vi "eserc_4_lettura.vi"() -> ()   [LabVIEW 2021]
uses:
  DMM4.lvlib
panel:
  out "CORRENTE":dbl[](array[numeric])=[2.0202, 2.0202, 2.0202, 2.0202, 2.0203, 2.0203, 2.0203, 2.0203, 2.0203, 2.0203, 2.0203, 2.0203, 2.0203, 2.0203, 2.0203, 2.0203, 2.0203, 2.0203, 2.0203, 2.0203, 2.0203, 2.0203, 2.0203, 2.0203, 2.0203, 2.0203, 2.0203, 2.0203, 2.0203, 2.0203, 2.0203, 2.0203, 2.0203, 2.0203, 2.0203, 2.0203, 2.0203, 2.0203, 2.0203, 2.0203, 2.0203, 2.0203, 2.0203, 2.0203, 2.0203, 2.0203, 2.0203, 2.0203, 2.0203, 2.0203, 2.0203, 2.0203, 2.0203, 2.0203, 2.0203, 2.0203, 2.0203, 2.0203, 2.0203, 2.0203, 2.0203, 2.0203, 2.0203, 2.0203, 2.0203, 2.0203, 2.0203, 2.0203, 2.0203, 2.0203, 2.0203, 2.0203, 2.0203, 2.0203, 2.0203, 2.0203, 2.0203, 2.0203, 2.0203, 2.0203, 2.0203, 2.0203, 2.0203, 2.0203, 2.0203, 2.0203, 2.0203, 2.0203, 2.0203, 2.0203, 2.0203, 2.0203, 2.0203, 2.0203, 2.0203, 2.0203, 2.0203, 2.0203, 2.0203, 2.0203]
  out "TENSIONE":dbl[](array[numeric])=[0.00906, 0.00906, 0.00906, 0.00906, 0.00906, 0.00906, 0.00906, 0.00906, 0.00906, 0.00906, 0.00906, 0.00906, 0.00906, 0.00906, 0.00906, 0.00906, 0.00906, 0.00906, 0.00906, 0.00906, 0.00906, 0.00906, 0.00906, 0.00906, 0.00906, 0.00906, 0.00906, 0.00906, 0.00906, 0.00906, 0.00906, 0.00906, 0.00906, 0.00905, 0.00905, 0.00905, 0.00906, 0.00906, 0.00906, 0.00906, 0.00905, 0.00905, 0.00905, 0.00906, 0.00906, 0.00906, 0.00906, 0.00906, 0.00906, 0.00906, 0.00905, 0.00905, 0.00905, 0.00905, 0.00906, 0.00905, 0.00906, 0.00906, 0.00906, 0.00906, 0.00905, 0.00906, 0.00906, 0.00906, 0.00906, 0.00906, 0.00905, 0.00905, 0.00905, 0.00905, 0.00906, 0.00906, 0.00906, 0.00906, 0.00906, 0.00905, 0.00905, 0.00906, 0.00905, 0.00905, 0.00905, 0.00905, 0.00905, 0.00905, 0.00905, 0.00905, 0.00905, 0.00905, 0.00905, 0.00906, 0.00905, 0.00905, 0.00905, 0.00905, 0.00905, 0.00906, 0.00905, 0.00905, 0.00905, 0.00906]
  in  "BOTTONE A":bool
  in  "BOTTONE V":bool
  out "error out 2":errorcluster
  out "Measure Value 2":string="+2.0203E+0\r\n"
  in  "Stop 2":bool
  out "Boolean 2":bool=TRUE
  in  "Detector Rate 2":u16(ring) items=["SLOW", "MID", "FAST"]
  in  "Manual Range 2":dbl=5.0 format="%#.9e"
  in  "Enable Auto Range 2":bool
  out "ID Return String 2":string="GWInstek,GDM8341,GEP843370,1.03\r\n"
  in  "Configure RS232 Baud Rate 2":u32(ring)=115200 items=["9600"=9600, "19200"=19200, "38400"=38400, "57600"=57600, "115200"=115200]
  in  "VISA resource name 2":refnum<visa-resource-name>="COM5"
  out "Boolean":bool=TRUE
  out "error out":errorcluster
  in  "Stop":bool
  out "Measure Value":string="+0.906E-2\r\n"
  in  "Detector Rate":u16(ring) items=["SLOW", "MID", "FAST"]
  in  "Manual Range":dbl format="%#.9e"
  in  "Enable Auto Range":bool=TRUE
  out "ID Return String":string="GWInstek,GDM8341,GEP843402,1.03\r\n"
  in  "Configure RS232 Baud Rate":u32(ring)=115200 items=["9600"=9600, "19200"=19200, "38400"=38400, "57600"=57600, "115200"=115200]
  in  "VISA resource name":refnum<visa-resource-name>="COM4"
  # "DC AMPERE"
  # "DMM Read DC Voltage"
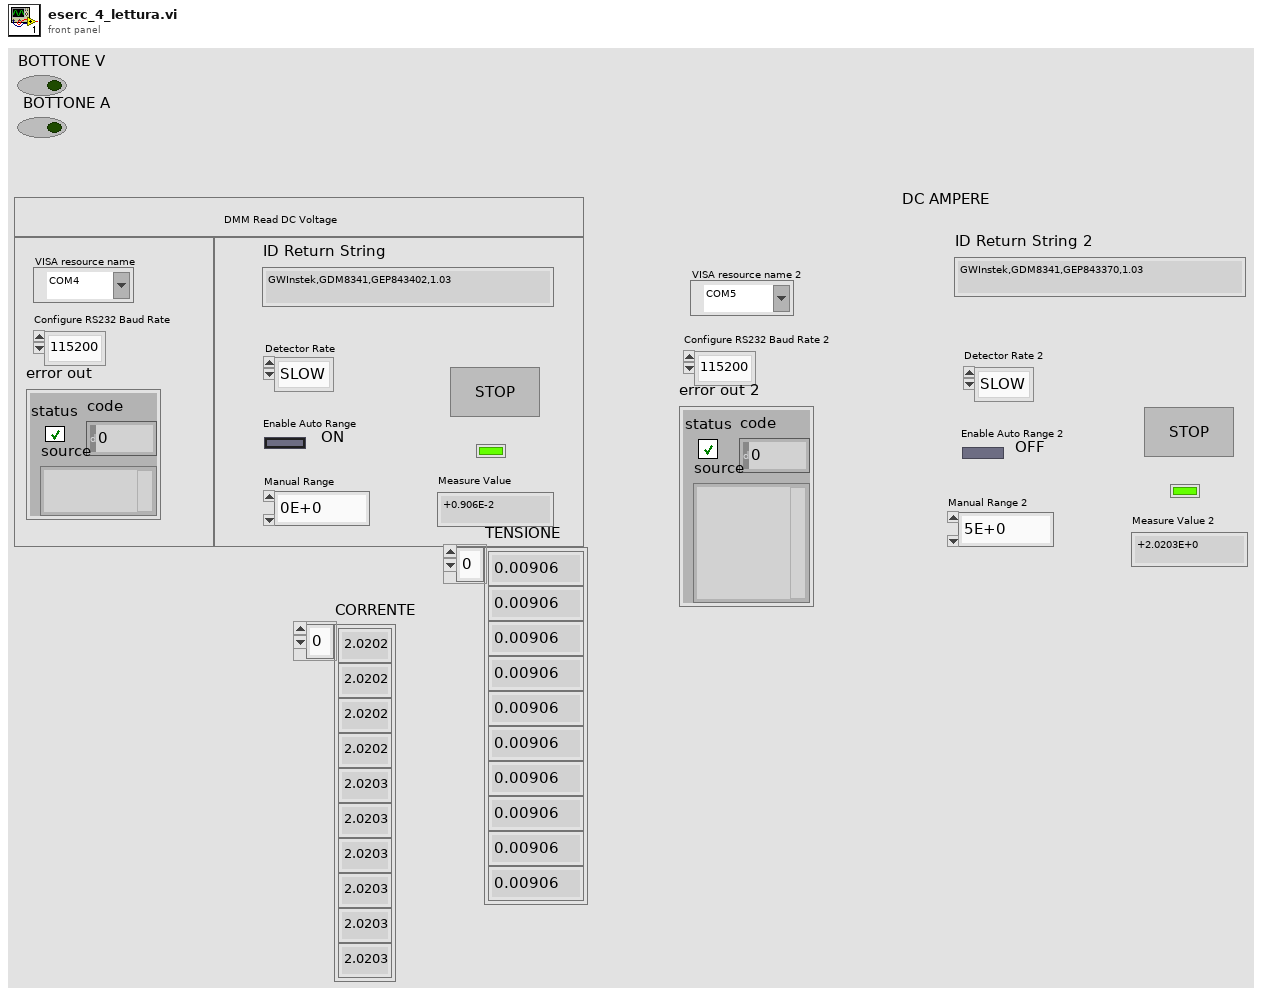
[diagram p1: front panel]
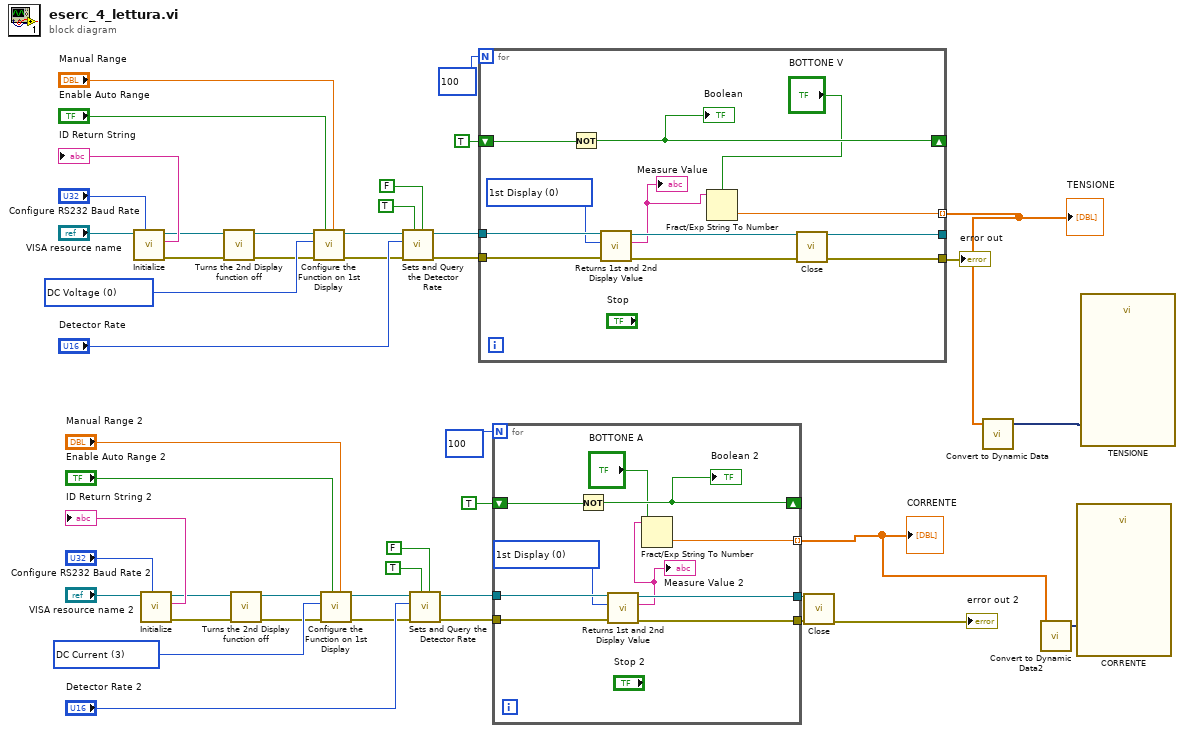
[diagram p0: block diagram]
diagram:
  w24 = u8 3 items=["DC Voltage", "AC Voltage", "DC+AC Voltage", "DC Current", "AC Current", "DC+AC Current", "2-Wire Resistance", "Frequency", "Period", "Continuity", "Diode", "Temperature", "Capacitance"] ("Function")
  w45 = u8 0 items=["DC Voltage", "AC Voltage", "DC+AC Voltage", "DC Current", "AC Current", "DC+AC Current", "2-Wire Resistance", "Frequency", "Period", "Continuity", "Diode", "Temperature", "Capacitance"] ("Function")
  n1 = call "Initialize.vi"("Configure RS232 Baud Rate"="Configure RS232 Baud Rate", "VISA resource name"="VISA resource name") -> ("error out"=w31:errorcluster, "ID Return String"=→"ID Return String":string, "VISA resource name out"=w32:refnum<visa-resource-name>)  [unwired: 6 in, 1 out]
  n2 = call "Initialize.vi"("Configure RS232 Baud Rate"="Configure RS232 Baud Rate 2", "VISA resource name"="VISA resource name 2") -> ("error out"=w10:errorcluster, "ID Return String"=→"ID Return String 2":string, "VISA resource name out"=w11:refnum<visa-resource-name>)  [unwired: 6 in, 1 out]
  n3 = call "Turns the 2nd Display function off.vi"("error in"=w31, "VISA resource name"=w32) -> ("error out"=w29:errorcluster, "VISA resource name out"=w30:refnum<visa-resource-name>)  [unwired: 8 in]
  n4 = call "Turns the 2nd Display function off.vi"("error in"=w10, "VISA resource name"=w11) -> ("error out"=w8:errorcluster, "VISA resource name out"=w9:refnum<visa-resource-name>)  [unwired: 8 in]
  n5 = call "Configure the Function on 1st Display .vi"("Manual Range"="Manual Range", "Enable Auto Range"="Enable Auto Range", "error in"=w29, "Function"=w45, "VISA resource name"=w30) -> ("error out"=w33:errorcluster, "VISA resource name out"=w34:refnum<visa-resource-name>)  [unwired: 5 in]
  n6 = call "Configure the Function on 1st Display .vi"("Manual Range"="Manual Range 2", "Enable Auto Range"="Enable Auto Range 2", "error in"=w8, "Function"=w24, "VISA resource name"=w9) -> ("error out"=w12:errorcluster, "VISA resource name out"=w13:refnum<visa-resource-name>)  [unwired: 5 in]
  n7 = call "Sets and Query the Detector Rate.vi"("Enable to Query"=FALSE, "Enable to Sets"=TRUE, "error in"=w33, "Detector Rate"="Detector Rate", "VISA resource name"=w34) -> ("error out"=w38:errorcluster, "VISA resource name out"=w39:refnum<visa-resource-name>)  [unwired: 4 in, 1 out]
  n8 = call "Sets and Query the Detector Rate.vi"("Enable to Query"=FALSE, "Enable to Sets"=TRUE, "error in"=w12, "Detector Rate"="Detector Rate 2", "VISA resource name"=w13) -> ("error out"=w17:errorcluster, "VISA resource name out"=w18:refnum<visa-resource-name>)  [unwired: 4 in, 1 out]
  n9 = for {
    N: 100 -> [_]
    tunnel: w39 -> [w58]
    tunnel: w38 -> [w57]
    tunnel: [w55] -> w37
    tunnel: [w54] -> w36
    shift-right: [w52] -> _
    shift-left: TRUE -> [w53]
    tunnel: [w49] -> w4 mode=indexing
    w56 = u16 0 items=["1st Display", "2nd Display", "1st & 2nd Display"] ("Sets to Display")
    n10 = Not(x=w53) -> (.not. x?=w52:bool)
    "Boolean" <- w52
    n11 = call "Returns 1st and 2nd Display Value.vi"("error in"=w57, "Sets to Display"=w56, "VISA resource name"=w58) -> ("error out"=w54:errorcluster, "Return the Value"=w51:string, "VISA resource name out"=w55:refnum<visa-resource-name>)  [unwired: 6 in]
    "Measure Value" <- w51
    n12 = Fract/Exp String To Number(use system decimal point (T)="BOTTONE V", string=w51) -> (number=w49:dbl)  [unwired: 2 in, 1 out]
  }
  "TENSIONE" <- w4
  n13 = for {
    N: 100 -> [_]
    tunnel: w18 -> [w68]
    tunnel: w17 -> [w67]
    tunnel: [w65] -> w16
    tunnel: [w64] -> w15
    shift-right: [w62] -> _
    shift-left: TRUE -> [w63]
    tunnel: [w59] -> w2 mode=indexing
    w66 = u16 0 items=["1st Display", "2nd Display", "1st & 2nd Display"] ("Sets to Display")
    n14 = Not(x=w63) -> (.not. x?=w62:bool)
    "Boolean 2" <- w62
    n15 = call "Returns 1st and 2nd Display Value.vi"("error in"=w67, "Sets to Display"=w66, "VISA resource name"=w68) -> ("error out"=w64:errorcluster, "Return the Value"=w61:string, "VISA resource name out"=w65:refnum<visa-resource-name>)  [unwired: 6 in]
    "Measure Value 2" <- w61
    n16 = Fract/Exp String To Number(use system decimal point (T)="BOTTONE A", string=w61) -> (number=w59:dbl)  [unwired: 2 in, 1 out]
  }
  "CORRENTE" <- w2
  n17 = call "Close.vi"("error in (no error)"=w36, "VISA resource name"=w37) -> ("error out"=→"error out":errorcluster)  [unwired: 9 in]
  n18 = call "Close.vi"("error in (no error)"=w15, "VISA resource name"=w16) -> ("error out"=→"error out 2":errorcluster)  [unwired: 9 in]
  n19 = call "Convert to Dynamic Data"("Array"=w4) -> ("Dynamic Data Type"=w3:dynamicdata)  [unwired: 3 in]
  n20 = call "Convert to Dynamic Data2"("Array"=w2) -> ("Dynamic Data Type"=w1:dynamicdata)  [unwired: 3 in]
  n21 = call "CORRENTE"("Signals"=w1) -> ()  [unwired: 16 in, 3 out]
  n22 = call "TENSIONE"("Signals"=w3) -> ()  [unwired: 16 in, 3 out]
